vi "Config_Infos.vi"() -> ()   [LabVIEW 2016]
panel:
  in  "xml_files_folder":string
  in  "dripline_info":string
  in  "service_name":string
  in  "COMport":i32
  in  "averaging_time":i32
  out "remove_processed_files":bool
  in  "wait_before_broadcasting":i32
  in  "broker":string
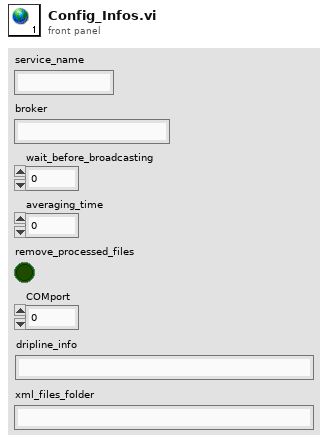
[diagram p1: front panel]
diagram:
